vi "LWXPS_PositionerCorrectorSR1ObserverAccelerationGet.vi"(0 "XPS Reference IN":refnum<k24>, 7 "Positioner Name":string, 11 "LabVIEW error IN":errorcluster) -> (3 "XPS Reference OUT":refnum<k24>, 4 "Returned error code":i32, 6 "Parameter A":dbl, 8 "Parameter B":dbl, 10 "Parameter C":dbl, 14 "LabVIEW error OUT":errorcluster, 15 "XPS Error String":string)   [LabVIEW 2014]
uses:
  D:/XPSQ8_LabView_Library/Development/Source/Dll/Newport.XPS.CommandInterface.dll
  Dll/Newport.XPS.CommandInterface.dll
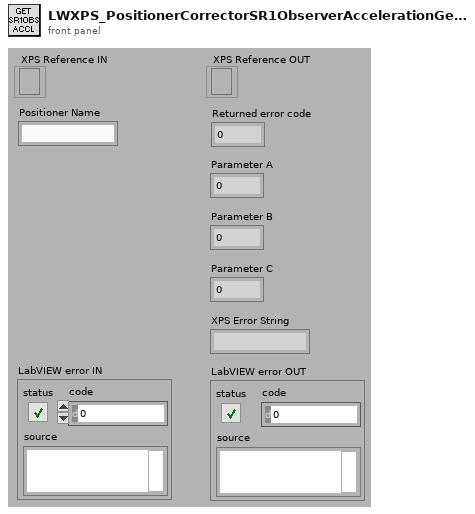
[diagram p1: front panel]
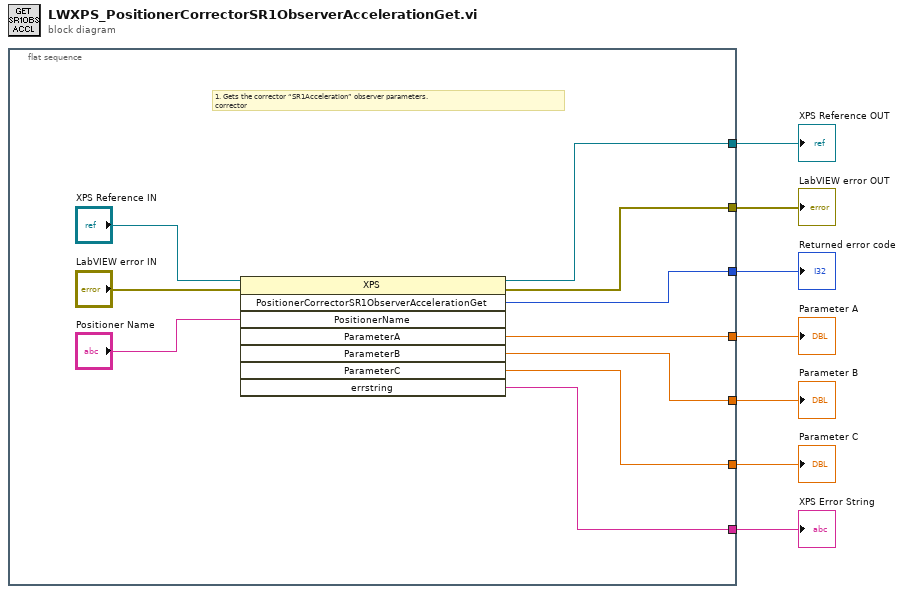
[diagram p0: block diagram]
diagram:
  n1 = flat-sequence {
    tunnel: [w15] -> w7
    tunnel: [w12] -> w6
    tunnel: [w16] -> w5
    tunnel: [w10] -> w3
    tunnel: [w11] -> w4
    tunnel: [w8] -> w1
    tunnel: [w9] -> w2
    frame #0 {
      # "1. Gets the corrector “SR1Acceleration” observer parameters.\ncorrector"
      n2 = invoke class="XPS" method="PositionerCorrectorSR1ObserverAccelerationGet"(reference="XPS Reference IN", error in="LabVIEW error IN", "PositionerName"="Positioner Name") -> (reference out=w15:refnum<k24>, error out=w12:errorcluster, "PositionerCorrectorSR1ObserverAccelerationGet"=w16:i32, "ParameterA"=w10:dbl, "ParameterB"=w11:dbl, "ParameterC"=w9:dbl, "errstring"=w8:string)  [unwired: 5 in, 1 out]
    }
  }
  "XPS Error String" <- w1
  "XPS Reference OUT" <- w7
  "LabVIEW error OUT" <- w6
  "Returned error code" <- w5
  "Parameter B" <- w4
  "Parameter A" <- w3
  "Parameter C" <- w2
